vi "Match value to time constant.vi"(11 "integer":i8) -> (3 "time constant":dbl[unit])   [LabVIEW 2009, in "SR830.lvlib"]
doc: "Takes an integer input (the value returned by the lock-in) and matches it to its corresponding time constant."
uses:
  time constants.ctl
  sr830/SR830.lvlib
panel:
  in  "Lock-in time constants":T1 items=["0"=1e-05, "1"=3e-05, "2"=0.0001, "3"=0.0003, "4"=0.001, "5"=0.003, "6"=0.01, "7"=0.03, "8"=0.1, "9"=0.3, "10"=1.0, "11"=3.0, "12"=10.0, "13"=30.0, "14"=100.0, "15"=300.0, "16"=1000.0, "17"=3000.0, "18"=10000.0, "19"=30000.0]
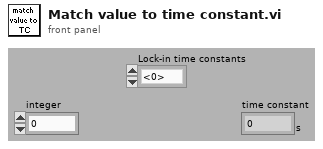
[diagram p1: front panel]
types:
  T1 = typedef "SR830.lvlib/time constants.ctl" = dbl
  T2 = typedef "LVStringsAndValuesArrayTypeDef.ctl" = cluster{"String":string, "Value":dbl}[]
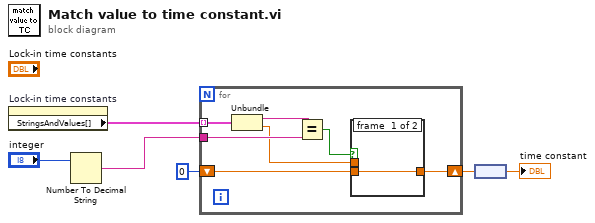
[diagram p0: block diagram]
diagram:
  n1 = property on="Lock-in time constants" class="Ring (strict)"() -> ("StringsAndValues[]"=w3:T2)  [unwired: 2 in, 2 out]
  n2 = Number To Decimal String(number="integer") -> (decimal integer string=w5:string)  [unwired: 1 out]
  n3 = for {
    tunnel: w3 -> [w9] mode=indexing
    tunnel: w5 -> [w13]
    shift-right: [w11] -> w1
    shift-left: 0 -> [w10]
    n4 = Unbundle(w9) -> ("String"=w8:string, "Value"=w7:dbl)
    n5 = Equal?(x=w8, y=w13) -> (x = y?=w12:bool)
    n6 = case shown="True" w12 {
      tunnel: [w14 w15] -> w11
      tunnel: w10 -> [w14 _]
      tunnel: w7 -> [_ w15]
      frame #0 {
      }
      frame #1 {
      }
    }
  }
  n7 = node(w1) -> (→"time constant":dbl[unit])
